vi "test_NoServicesRegistered_InvalidRegisterRequests_Error.vi"() -> (6 "pass":bool, 8 "result":string, 15 "error out":errorcluster)   [LabVIEW 2020]
uses:
  Runtime/MeasurementLink Discovery Client/RPC Messages/ni_measurementlink_discovery_v1_RegisterServiceRequest.ctl
  Runtime/MeasurementLink Discovery Client/RPC Messages/ni_measurementlink_discovery_v1_ServiceDescriptor.ctl
  Runtime/MeasurementLink Discovery Client/RPC Messages/ni_measurementlink_discovery_v1_ServiceLocation.ctl
  <vilib>/ErrorRing/Error Ring.xnode
  Runtime/MeasurementLink Discovery Client/MeasurementLink Discovery Client.lvlib
panel:
  # "Test assumes discovery service has already been started."
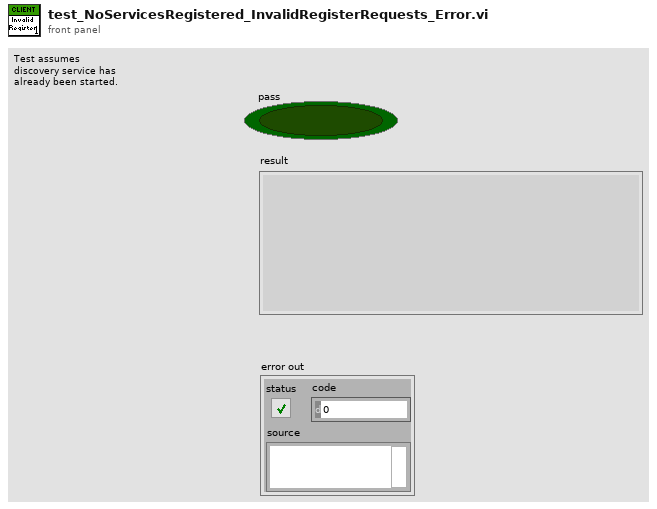
[diagram p1: front panel]
types:
  T1 = typedef "MeasurementLink Discovery Client.lvlib/ni_measurementlink_discovery_v1_RegisterServiceRequest.ctl" = cluster{"service_description":T2, "location":T3}
  T2 = typedef "MeasurementLink Discovery Client.lvlib/ni_measurementlink_discovery_v1_ServiceDescriptor.ctl" = cluster{"display_name":string, "description_url":string, "provided_interfaces":string[], "service_class":string}
  T3 = typedef "MeasurementLink Discovery Client.lvlib/ni_measurementlink_discovery_v1_ServiceLocation.ctl" = cluster{"location":string, "insecure_port":string, "ssl_authenticated_port":string}
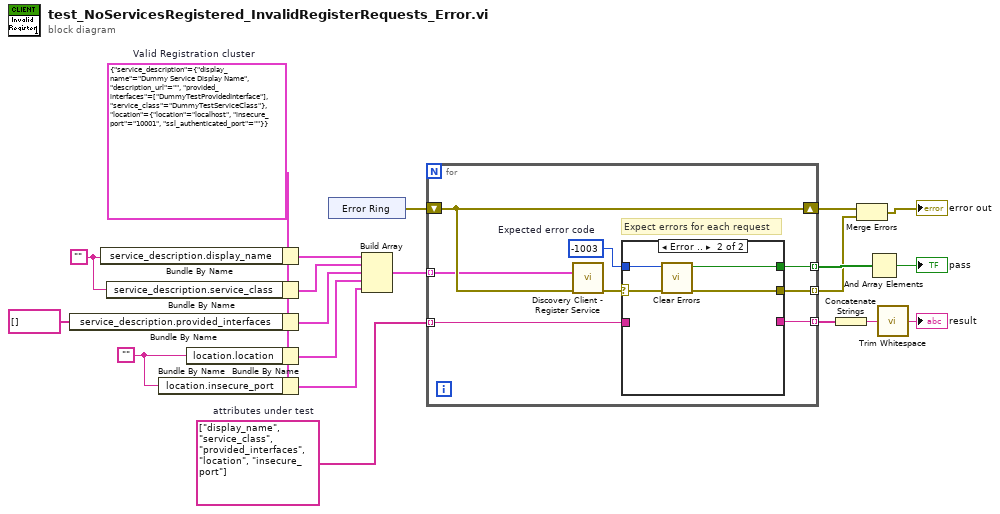
[diagram p0: block diagram]
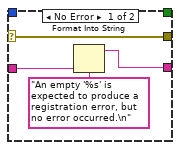
[diagram p2: hidden frame]
diagram:
  w4 = string[] ["display_name", "service_class", "provided_interfaces", "location", "insecure_port"]  # attributes under test
  w10 = ""
  w15 = ""
  w9 = T1 {"service_description"={"display_name"="Dummy Service Display Name", "description_url"="", "provided_interfaces"=["DummyTestProvidedInterface"], "service_class"="DummyTestServiceClass"}, "location"={"location"="localhost", "insecure_port"="10001", "ssl_authenticated_port"=""}}  # Valid Registration cluster
  n1 = Bundle By Name(cluster=w9, "service_description.provided_interfaces"=string[] []) -> (w13:T1)
  n2 = Bundle By Name(cluster=w9, "service_description.display_name"=w15) -> (w16:T1)
  n3 = Bundle By Name(cluster=w9, "service_description.service_class"=w15) -> (w14:T1)
  n4 = Bundle By Name(cluster=w9, "location.insecure_port"=w10) -> (w8:T1)
  n5 = Bundle By Name(cluster=w9, "location.location"=w10) -> (w11:T1)
  n6 = xnode "Error Ring"() -> ("error out"=w18:errorcluster)
  n7 = Build Array(w16, w14, w13, w11, w8) -> (w17:T1[])
  n8 = for {
    tunnel: [w26] -> w19 mode=indexing
    tunnel: w17 -> [w27] mode=indexing
    shift-right: [w28] -> w7
    shift-left: w18 -> [w28]
    tunnel: [w25] -> w5 mode=indexing
    tunnel: w4 -> [w22] mode=indexing
    tunnel: [w21] -> w3 mode=indexing
    w24 = -1003  # Expected error code
    # "Expect errors for each request"
    n9 = call "Discovery Client - Register Service.vi"("Request Data"=w27, "error in (no error)"=w28) -> ("error out"=w23:errorcluster)  [unwired: 12 in, 1 out]
    n10 = case shown="Error .." w23 {
      selector: w23 -> [w32 w33]
      tunnel: [_ w36] -> w26
      tunnel: [w32 w35] -> w25
      tunnel: w24 -> [_ w34]
      tunnel: w22 -> [w31 _]
      tunnel: [w29 _] -> w21
      frame No Error {
        n11 = Format Into String(format string="An empty '%s' is expected to produce a registration error, but no error occurred.\n", w31) -> (resulting string=w29:string)  [unwired: 2 in, 1 out]
      }
      frame Error {
        n12 = call <vilib>:"Clear Errors.vi"("error in (no error)"=w33, "specific error code to clear (0: all)"=w34) -> ("error out"=w35:errorcluster, "specific error cleared?"=w36:bool)  [unwired: 4 in]
      }
    }
  }
  n13 = Concatenate Strings(w3) -> (w2:string)
  n14 = Merge Errors(w7, w5) -> (→"error out":errorcluster)
  n15 = And Array Elements(Boolean array=w19) -> (logical AND=→"pass":bool)
  n16 = call <vilib>:"Trim Whitespace.vi"("string"=w2) -> ("trimmed string"=→"result":string)  [unwired: 1 in]
